vi "monitor scan logic.vi"(0 "Array IN":T4[](array[typedef]), 1 "monitor action":T3 caption="aaa", 2 "init":bool=TRUE, 5 "freq IN":dbl[](array[numeric]), 7 "Magn Field (T)":dbl, 9 "gamma IN":dbl[](array[numeric]), 11 "monitor state":T2={"header - gamma"=[], "header - frequency"=[], "# of peaks"=28, "peaks OK"=TRUE}, 12 "scan monitor control IN":T1={"gamma acc. frac. - min "=0.7, "gamma acc frac.. - max"=1.3, "peak acc. fraction (af)"=0.1, "min peak acc. window (kHz)"=0.1, "use"=enum."fraction", "abs gamma min(kHz)"=0.03, "abs gamma max(kHz)"=10.0, "# points"=0, "gamma-factor (fa)"=10.0, "interpolate"=enum."last", "init"=FALSE, "Unique strike parameters"=FALSE, "max peak acc. window (kHz)"=10.0, "spacing factor"=3.0, "iterate #"=1, "overwrite ctl?"=TRUE, "write _m files?"=FALSE, "max slope (kHz/sweep)"=0.1, "funnel state"=enum."funnel open"}, 13 "Sweep folder path":path=path "E:/data/Ultrasound/Experiment/ProbeTest/Probe10/Hg1201-350CO2-3b-96K/sweep2", 14 "temperature":dbl=309.595) -> (4 "Array OUT":T4[](array[typedef]), 6 "freq OUT":dbl[](array[numeric]), 10 "gamma OUT":dbl[](array[numeric]), 15 "monitor state OUT":T2={"header - gamma"=[], "header - frequency"=[], "# of peaks"=28, "peaks OK"=TRUE})   [LabVIEW 2015]
uses:
  peak monitor ctl - V2.ctl
  interpolation state - real.ctl
  parameters -- scan monitor control.ctl
  monitor action.ctl
  monitor state.ctl
  ctl -- name dispatcher -- action.ctl
  next chunk read-write PID -- action.ctl
  agregator -- action.ctl
  Q - not nan -- real.vi
  ctl -- name dispatcher.vi
  file -- 9w path.vi
  array -- find index - real.vi
  array -- interpolate -- i.vi
  Q - not nan -- integer.vi
  linear interpolation - real.vi
  <vilib>/gmath/function.llb/Binomial Coefficient.vi
  <vilib>/Utility/file.llb/Write To Spreadsheet File.vi
  <vilib>/Utility/file.llb/Write To Spreadsheet File (string).vi
  <vilib>/Utility/libraryn.llb/Check if File or Folder Exists.vi
  parse -- get list of matches -- numbers.vi
  parse -- find first line.vi
  file -- read list of lines.vi
panel:
  out "scan monitor control OUT":T1={"gamma acc. frac. - min "=0.7, "gamma acc frac.. - max"=1.3, "peak acc. fraction (af)"=0.1, "min peak acc. window (kHz)"=0.1, "use"=enum."fraction", "abs gamma min(kHz)"=0.03, "abs gamma max(kHz)"=10.0, "# points"=0, "gamma-factor (fa)"=10.0, "interpolate"=enum."last", "init"=FALSE, "Unique strike parameters"=FALSE, "max peak acc. window (kHz)"=10.0, "spacing factor"=3.0, "iterate #"=1, "overwrite ctl?"=TRUE, "write _m files?"=FALSE, "max slope (kHz/sweep)"=0.1, "funnel state"=enum."funnel open"}
  in  "Boolean":bool=TRUE
  # "three strikes"
  # "search window"
  # "linear extrapolation"
  # "three strikes"
  # "search window"
  # "linear extrapolation"
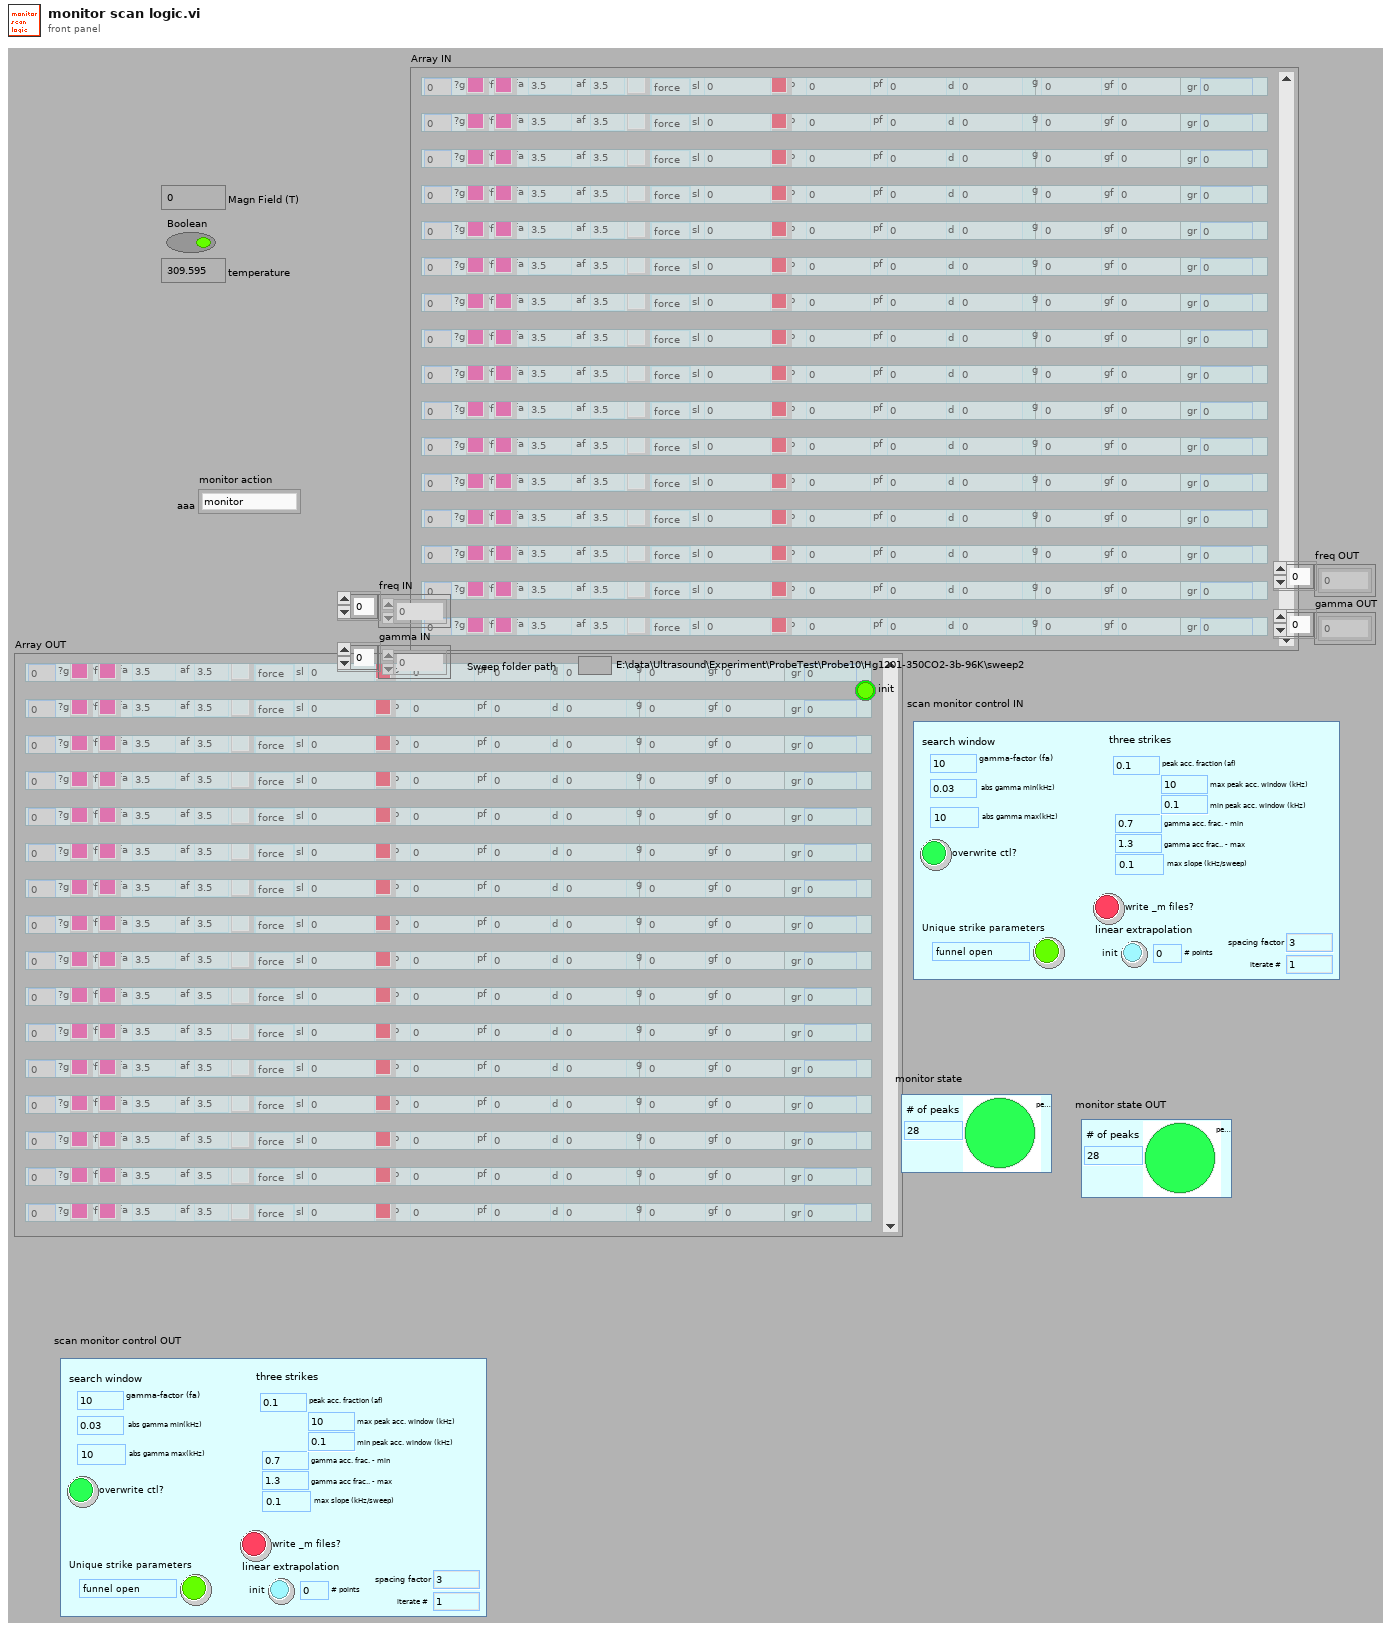
[diagram p1: front panel]
types:
  T1 = typedef "parameters -- scan monitor control.ctl" = cluster{"gamma acc. frac. - min ":dbl, "gamma acc frac.. - max":dbl, "peak acc. fraction (af)":dbl, "min peak acc. window (kHz)":dbl, "use":enum16{"window", "fraction"}, "abs gamma min(kHz)":dbl, "abs gamma max(kHz)":dbl, "# points":i32, "gamma-factor (fa)":dbl, "interpolate":enum16{"line", "last"}, "init":bool, "Unique strike parameters":bool, "max peak acc. window (kHz)":dbl, "spacing factor":dbl, "iterate #":i32, "overwrite ctl?":bool, "write _m files?":bool, "max slope (kHz/sweep)":dbl, "funnel state":enum16{"funnel open", "funnel closed"}}
  T2 = typedef "monitor state.ctl" = cluster{"header - gamma":string[], "header - frequency":string[], "# of peaks":i32, "peaks OK":bool}
  T3 = typedef "monitor action.ctl" = enum16{"monitor", "interpolate", "global", "read", "overwrite", "write m file", "nothing", "eeee"}
  T4 = typedef "peak monitor ctl - V2.ctl" = cluster{"delta":dbl, "gamma":dbl, "exp":dbl, "found?":bool, "found":dbl, "gamma found":dbl, "init linear":bool, "interpolate":enum16{"line", "force"}, "gamma-factor":dbl, "slope":dbl, "update freq?":bool, "update gamma?":bool, "acc factor":dbl, "linear interpolation state":T5, "ind":dbl, "gamma ratio":dbl, "gamma off limit?":bool, "freq off limit?":bool}
  T5 = typedef "interpolation state - real.ctl" = cluster{"requested size":i32, "Array":dbl[], "actual number of elements":i32}
  T6 = typedef "ctl -- name dispatcher -- action.ctl" = enum16{"peak frequency", "peak frequency DUMP", "peak gamma DUMP", "peak gamma", "peak frequency TEST", "peak gamma TEST", "ultrasonic power", "time in gamma", "set temperature ", "set temperature timer", "peak default gamma", "last scan file", "peak freq gamma TEST", "peak NAMES", "errors", "P_I_D", "P", "I", "D", "power vs time", "power vs time TIMER", "void", "power log", "set temperature - SINE", "itc ltc log", "peak - time in gamma"}
  T7 = typedef "agregator -- action.ctl" = enum16{"append", "interpolate", "empty!", "force"}
  T8 = typedef "next chunk read-write PID -- action.ctl" = enum16{"read", "interpolate", "append col", "write", "write PID col", "append PID col", "interpolate - bezier"}
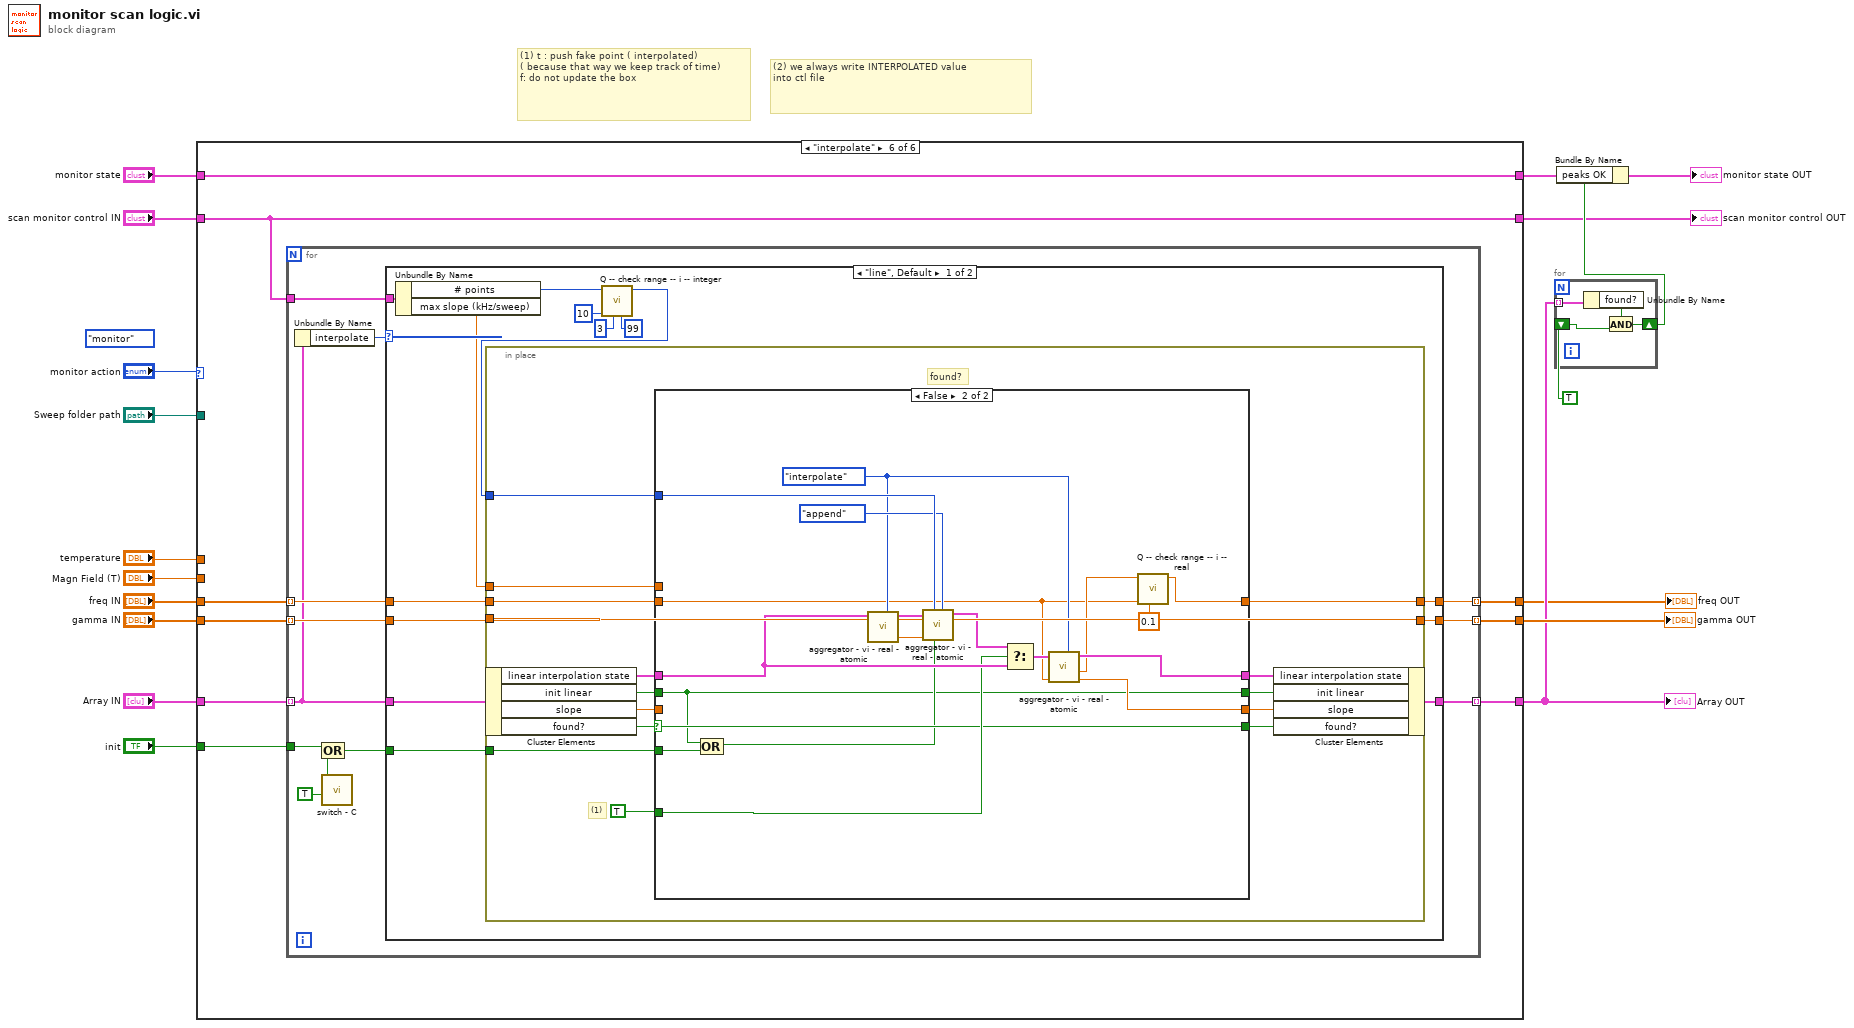
[diagram p0: block diagram]
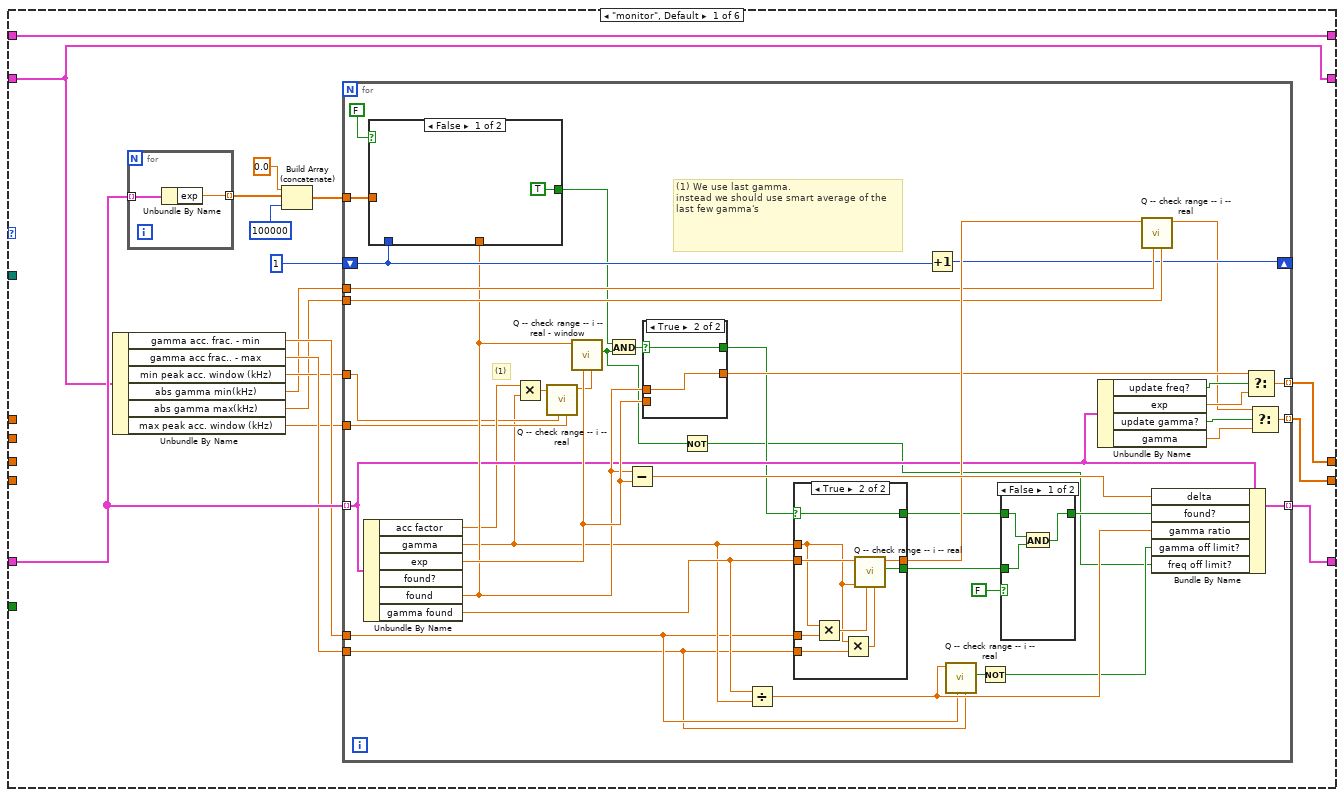
[diagram p2: hidden frame]
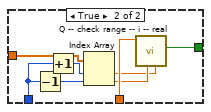
[diagram p3: hidden frame]
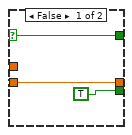
[diagram p6: hidden frame]
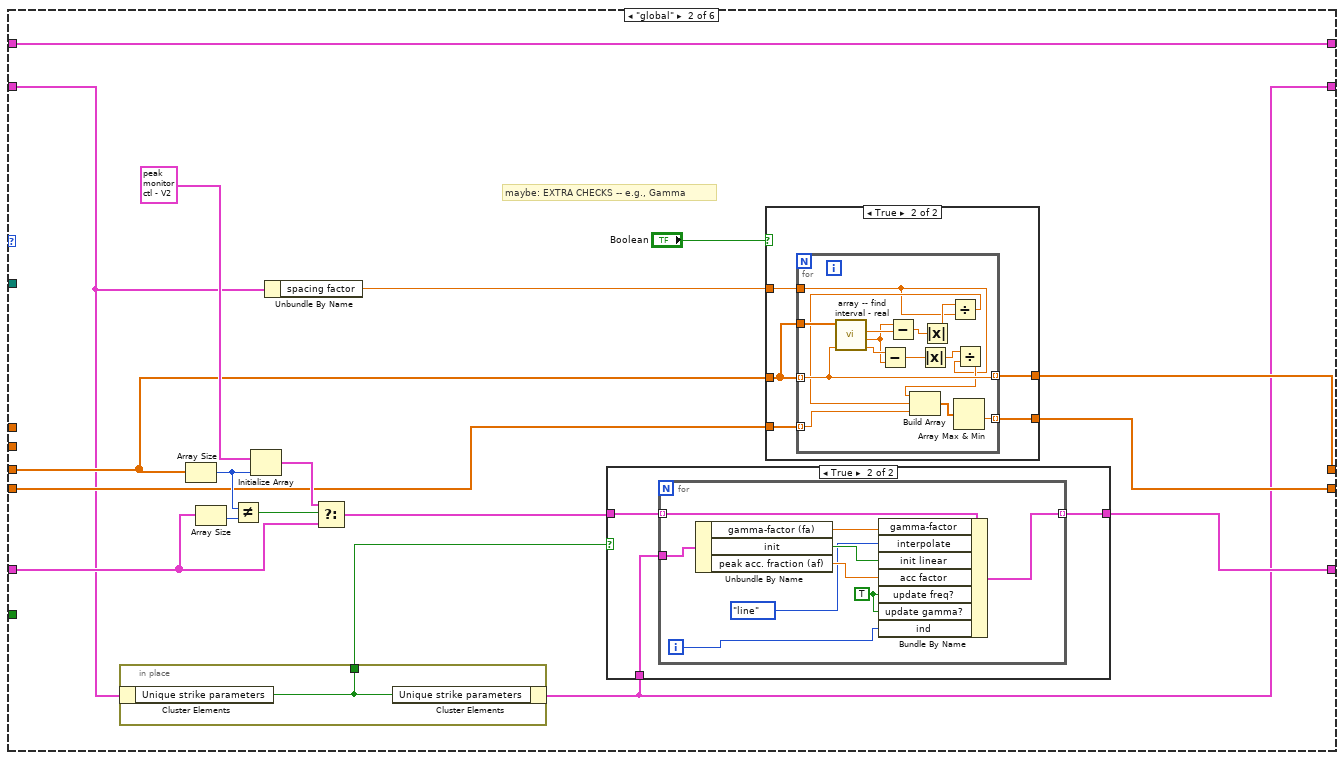
[diagram p7: hidden frame]
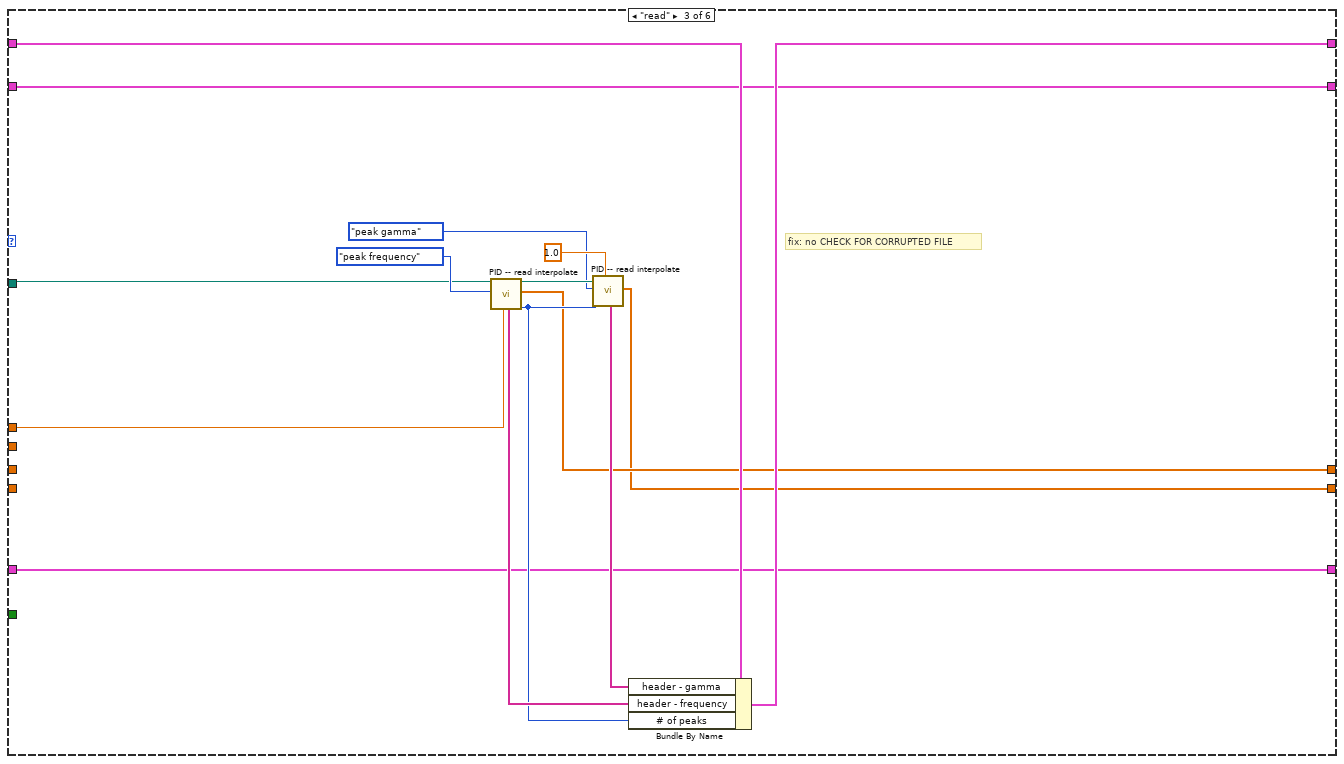
[diagram p10: hidden frame]
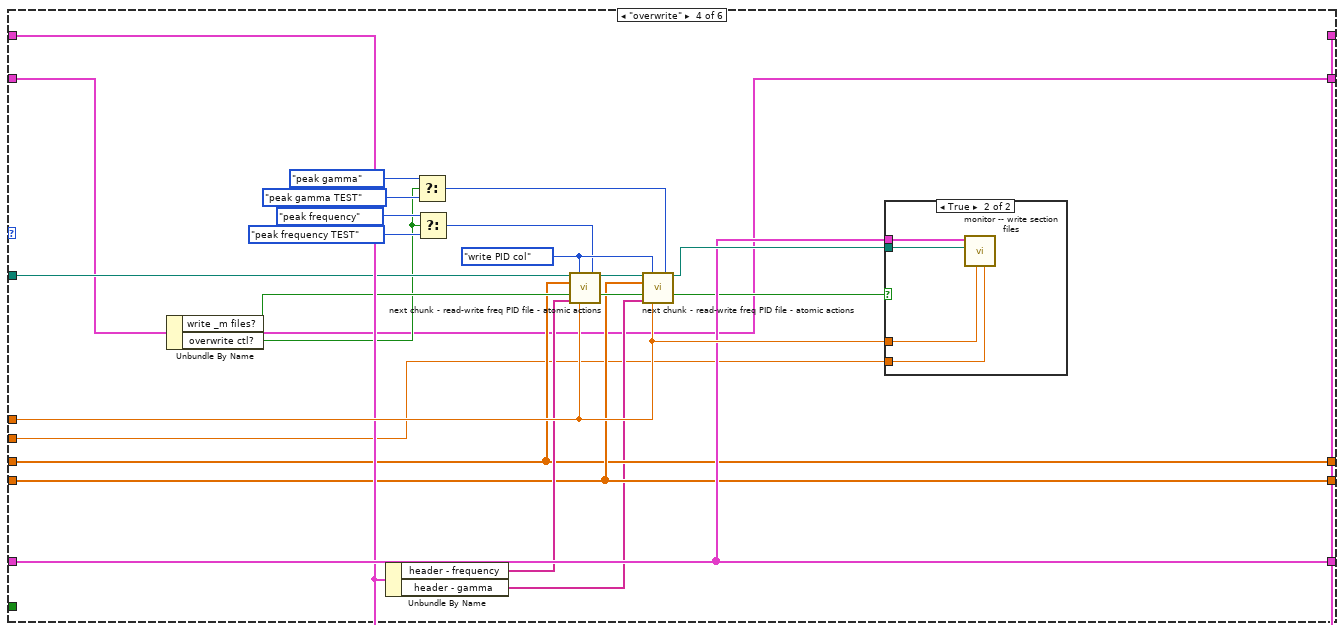
[diagram p11: hidden frame]
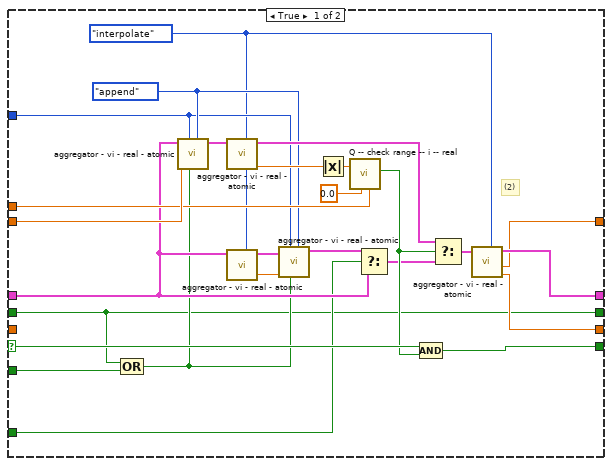
[diagram p14: hidden frame]
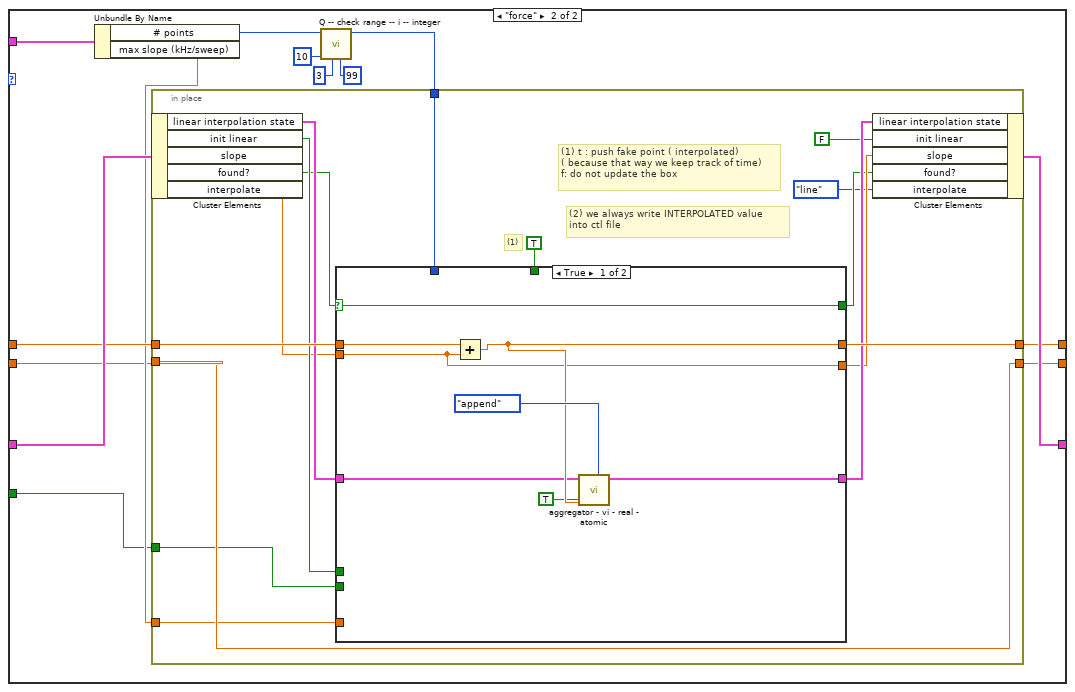
[diagram p15: hidden frame]
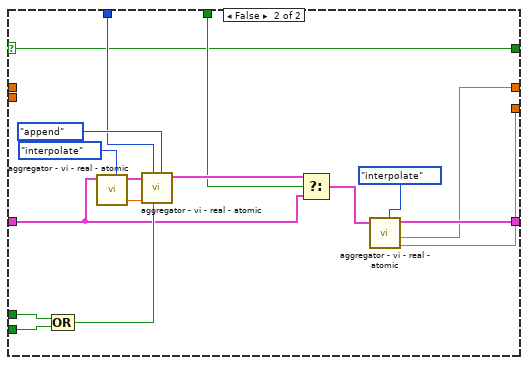
[diagram p16: hidden frame]
diagram:
  (unwired) monitor_action."monitor" ("monitor action")
  # "(2) we always write INTERPOLATED value \ninto ctl file"
  # "(1) t : push fake point ( interpolated) \n( because that way we keep track of time)\nf: do not update the box"
  n1 = case shown="\"interpolate\"" "monitor action" {
    tunnel: "scan monitor control IN" -> [w19 w109 w162 w177 w202 w207]
    tunnel: [w35 w115 w164 w180 w205 w214] -> w2
    tunnel: [w34 w114 w163 w181 w204 w212] -> w17
    tunnel: "Array IN" -> [w33 w119 w165 w187 w206 w215]
    tunnel: [w32 w125 w165 w187 w206 w210] -> w14
    tunnel: "freq IN" -> [_ w117 _ w180 w205 w213]
    tunnel: "gamma IN" -> [_ w116 _ w181 w204 w211]
    tunnel: "init" -> [_ _ _ _ _ w209]
    tunnel: "Sweep folder path" -> [_ _ w173 w184 _ _]
    tunnel: "temperature" -> [_ _ w172 w188 _ _]
    tunnel: "monitor state" -> [w20 w111 w170 w186 w203 w208]
    tunnel: [w20 w111 w167 w186 w203 w208] -> w5
    tunnel: "Magn Field (T)" -> [_ _ _ w178 _ _]
    tunnel: [w19 w108 w162 w177 w202 w207] -> w1
    frame "monitor", Default {
      n2 = Unbundle By Name(w19) -> ("gamma acc. frac. - min"=w31:dbl, "gamma acc frac.. - max"=w30:dbl, "min peak acc. window (kHz)"=w29:dbl, "abs gamma min(kHz)"=w28:dbl, "abs gamma max(kHz)"=w27:dbl, "max peak acc. window (kHz)"=w21:dbl)
      n3 = for {
        tunnel: w33 -> [w37] mode=indexing
        tunnel: [w36] -> w26 mode=indexing
        n4 = Unbundle By Name(w37) -> ("exp"=w36:dbl)
      }
      n5 = Build Array (concatenate)(0.0, w26, 100000) -> (w22:dbl[])
      n6 = for {
        tunnel: w33 -> [w66] mode=indexing
        tunnel: [w78] -> w32 mode=indexing
        tunnel: [w59] -> w34 mode=indexing
        tunnel: [w58] -> w35 mode=indexing
        tunnel: w31 -> [w44]
        tunnel: w30 -> [w43]
        tunnel: w29 -> [w56]
        tunnel: w28 -> [w75]
        tunnel: w27 -> [w74]
        shift-right: [w73] -> _
        shift-left: 1 -> [w72]
        tunnel: w22 -> [w71]
        tunnel: w21 -> [w55]
        # "(1)"
        # "(1) We use last gamma.\ninstead we should use smart average of the last few gamma's"
        n7 = Unbundle By Name(w66) -> ("acc factor"=w57:dbl, "gamma"=w46:dbl, "exp"=w69:dbl, "found"=w68:dbl, "gamma found"=w47:dbl)  [unwired: 1 out]
        n8 = case shown="False" FALSE ("in range?") {
          tunnel: w72 -> [_ w87]
          tunnel: w71 -> [_ w84]
          tunnel: w68 -> [_ w83]
          tunnel: [TRUE ("in range?") w80] -> w67
          frame False {
          }
          frame True {
            n9 = Decrement(x=w87) -> (x-1=w85:i32)
            n10 = Increment(x=w87) -> (x+1=w86:i32)
            n11 = Index Array(array=w84, index #1=w86, index #2=w85) -> (element #1=w81:dbl, element #2=w82:dbl)
            n12 = call "Q -- check range -- i -- real.vi"("upper"=w81, "lower"=w82, "number"=w83) -> ("in range?"=w80:bool)  [unwired: 6 in, 2 out]
          }
        }
        n13 = Multiply(x=w57, y=w46) -> (x*y=w54:dbl)
        n14 = call "Q -- check range -- i -- real.vi"("upper"=w55, "lower"=w56, "number"=w54) -> ("number in range"=w53:dbl)  [unwired: 6 in, 2 out]
        n15 = call "Q -- check range -- i -- real - window.vi"("window"=w53, "center"=w69, "number"=w68) -> ("in range?"=w40:bool)  [unwired: 6 in, 2 out]
        n16 = And(x=w67, y=w40) -> (x .and. y?=w70:bool)
        n17 = Subtract(x=w68, y=w69) -> (x-y=w77:dbl)
        n18 = case shown="True" w70 {
          selector: w70 -> [w92 w95]
          tunnel: [w92 w95] -> w52
          tunnel: [w93 w94] -> w64
          tunnel: w68 -> [_ w94]
          tunnel: w69 -> [w93 _]
          frame False {
          }
          frame True {
          }
        }
        n19 = Not(x=w40) -> (.not. x?=w39:bool)
        n20 = Divide(x=w47, y=w46) -> (x/y=w45:dbl)
        n21 = case shown="True" w52 {
          selector: w52 -> [w96 w99]
          tunnel: w47 -> [_ w107]
          tunnel: w46 -> [w98 w105]
          tunnel: [w98 w103] -> w76
          tunnel: w44 -> [_ w102]
          tunnel: w43 -> [_ w101]
          tunnel: [TRUE w100] -> w48
          tunnel: [w96 w99] -> w49
          frame False {
          }
          frame True {
            n22 = Multiply(x=w105, y=w102) -> (x*y=w106:dbl)
            n23 = Multiply(x=w105, y=w101) -> (x*y=w104:dbl)
            n24 = call "Q -- check range -- i -- real.vi"("upper"=w104, "lower"=w106, "default"=w105, "number"=w107) -> ("in range?"=w100:bool, "number in range"=w103:dbl)  [unwired: 5 in, 1 out]
          }
        }
        n25 = Increment(x=w72) -> (x+1=w73:i32)
        n26 = call "Q -- check range -- i -- real.vi"("upper"=w43, "lower"=w44, "number"=w45) -> ("in range?"=w42:bool)  [unwired: 6 in, 2 out]
        n27 = Not(x=w42) -> (.not. x?=w41:bool)
        n28 = case shown="False" FALSE {
          tunnel: [w88 w91] -> w50
          tunnel: w49 -> [w89 w91]
          tunnel: w48 -> [w90 _]
          frame False {
            n29 = And(x=w89, y=w90) -> (x .and. y?=w88:bool)
          }
          frame True {
          }
        }
        n30 = Unbundle By Name(w66) -> ("update freq?"=w65:bool, "exp"=w63:dbl, "update gamma?"=w62:bool, "gamma"=w60:dbl)
        n31 = call "Q -- check range -- i -- real.vi"("upper"=w74, "lower"=w75, "number"=w76) -> ("number in range"=w61:dbl)  [unwired: 6 in, 2 out]
        n32 = Bundle By Name(cluster=w66, "delta"=w77, "found?"=w50, "gamma ratio"=w45, "gamma off limit?"=w41, "freq off limit?"=w39) -> (w78:T4)
        n33 = Select(t=w64, s=w65, f=w63) -> (s? t:f=w58:dbl)
        n34 = Select(t=w61, s=w62, f=w60) -> (s? t:f=w59:dbl)
      }
    }
    frame "global" {
      # "maybe: EXTRA CHECKS -- e.g., Gamma"
      n35 = in-place {
        in-place-border: [w126] -> w110
        n36 = in-place-cluster #1(w109) -> ("Unique strike parameters"=w126:bool)
        n37 = in-place-cluster #1("Unique strike parameters"=w126) -> (w108:T1)
      }
      n38 = Array Size(array=w117) -> (size(s)=w123:i32)
      n39 = Array Size(array=w119) -> (size(s)=w124:i32)
      n40 = Not Equal?(x=w123, y=w124) -> (x != y?=w121:bool)
      n41 = Initialize Array(T4 {"delta"=0.0, "gamma"=0.0, "exp"=0.0, "found?"=FALSE, "found"=0.0, "gamma found"=0.0, "init linear"=FALSE, "interpolate"=enum."line", "gamma-factor"=0.0, "slope"=0.0, "update freq?"=FALSE, "update gamma?"=FALSE, "acc factor"=0.0, "linear interpolation state"={"requested size"=0, "Array"=[], "actual number of elements"=0}, "ind"=0.0, "gamma ratio"=0.0, "gamma off limit?"=FALSE, "freq off limit?"=FALSE} ("output cluster"), w123) -> (w120:T4[])
      n42 = Unbundle By Name(w109) -> ("spacing factor"=w112:dbl)
      n43 = Select(t=w120, s=w121, f=w119) -> (s? t:f=w118:T4[])
      n44 = case shown="True" w110 {
        tunnel: w118 -> [w149 w152]
        tunnel: [w149 w150] -> w125
        tunnel: w108 -> [_ w151]
        frame False {
        }
        frame True {
          n45 = for {
            tunnel: w152 -> [w156] mode=indexing
            tunnel: [w161] -> w150 mode=indexing
            tunnel: w151 -> [w160]
            i -> [w154]
            w155 = TRUE ("update freq?")
            n46 = Unbundle By Name(w160) -> ("gamma-factor (fa)"=w159:dbl, "init"=w158:bool, "peak acc. fraction (af)"=w157:dbl)
            n47 = Bundle By Name(cluster=w156, "gamma-factor"=w159, "interpolate"=enum16{"line", "force"}."line", "init linear"=w158, "acc factor"=w157, "update freq?"=w155, "update gamma?"=w155, "ind"=w154) -> (w161:T4)
          }
        }
      }
      n48 = case shown="True" "Boolean" {
        tunnel: w117 -> [w128 w133]
        tunnel: w116 -> [w127 w132]
        tunnel: [w128 w131] -> w115
        tunnel: [w127 w130] -> w114
        tunnel: w112 -> [_ w129]
        frame False {
        }
        frame True {
          n49 = for {
            tunnel: w133 -> [w144] mode=indexing
            tunnel: w133 -> [w148]
            tunnel: w132 -> [w141] mode=indexing
            tunnel: [w144] -> w131 mode=indexing
            tunnel: [w135] -> w130 mode=indexing
            tunnel: w129 -> [w134]
            n50 = call "array -- find interval - real.vi"("number"=w144, "array"=w148) -> ("omega plus (kHz)"=w146:dbl, "omega zero (kHz)"=w145:dbl, "omega minus (kHz)"=w147:dbl)  [unwired: 4 in, 3 out]
            n51 = Subtract(x=w146, y=w145) -> (x-y=w142:dbl)
            n52 = Subtract(x=w145, y=w147) -> (x-y=w143:dbl)
            n53 = Absolute Value(x=w142) -> (abs(x)=w139:dbl)
            n54 = Absolute Value(x=w143) -> (abs(x)=w140:dbl)
            n55 = Divide(x=w140, y=w134) -> (x/y=w137:dbl)
            n56 = Divide(x=w139, y=w134) -> (x/y=w138:dbl)
            n57 = Build Array(w138, w137, w141) -> (w136:dbl[])
            n58 = Array Max & Min(array=w136) -> (min value=w135:dbl)  [unwired: 3 out]
          }
        }
      }
    }
    frame "read" {
      # "fix: no CHECK FOR CORRUPTED FILE"
      n59 = call "PID -- read interpolate.vi"("sweep folder path"=w173, "ctl PID file IN"=ctl_--_name_dispatcher_--_action."peak frequency" ("ctl name dispatch"), "temperature"=w172) -> ("header"=w168:string[], "sweep folder path out"=w175:path, "PID freq"=w164:dbl[], "length out"=w166:i32)  [unwired: 11 in, 2 out]
      n60 = call "PID -- read interpolate.vi"("sweep folder path"=w175, "ctl PID file IN"=ctl_--_name_dispatcher_--_action."peak gamma" ("ctl name dispatch"), "length"=w166, "default"=1.0 ("element")) -> ("header"=w169:string[], "PID freq"=w163:dbl[])  [unwired: 10 in, 4 out]
      n61 = Bundle By Name(cluster=w170, "header - gamma"=w169, "header - frequency"=w168, "# of peaks"=w166) -> (w167:T2)
    }
    frame "overwrite" {
      w196 = next_chunk_read-write_PID_--_action."write PID col" ("PID action")
      n62 = Unbundle By Name(w177) -> ("write _m files?"=w183:bool, "overwrite ctl?"=w182:bool)
      n63 = Unbundle By Name(w186) -> ("header - frequency"=w185:string[], "header - gamma"=w179:string[])
      n64 = Select(t=ctl_--_name_dispatcher_--_action."peak gamma" ("ctl name dispatch"), s=w182, f=ctl_--_name_dispatcher_--_action."peak gamma TEST" ("ctl name dispatch")) -> (s? t:f=w195:T6)
      n65 = Select(t=ctl_--_name_dispatcher_--_action."peak frequency" ("ctl name dispatch"), s=w182, f=ctl_--_name_dispatcher_--_action."peak frequency TEST" ("ctl name dispatch")) -> (s? t:f=w194:T6)
      n66 = call "next chunk - read-write freq PID file - atomic actions .vi"("sweep folder path"=w184, "PID action"=w196, "ctl kind OUT"=w194, "PID freq IN"=w180, "header IN"=w185, "temperature"=w188) -> ("sweep folder path out"=w197:path)  [unwired: 5 in, 4 out]
      n67 = call "next chunk - read-write freq PID file - atomic actions .vi"("sweep folder path"=w197, "PID action"=w196, "ctl kind OUT"=w195, "PID freq IN"=w181, "header IN"=w179, "temperature"=w188) -> ("sweep folder path out"=w193:path)  [unwired: 5 in, 4 out]
      n68 = case shown="True" w183 {
        tunnel: w193 -> [_ w201]
        tunnel: w187 -> [_ w200]
        tunnel: w188 -> [_ w199]
        tunnel: w178 -> [_ w198]
        frame False {
        }
        frame True {
          n69 = call "monitor -- write section files.vi"("Magn Field (T)"=w198, "temperature"=w199, "Sweep folder path"=w201, "Array"=w200) -> ()  [unwired: 8 in]
        }
      }
    }
    frame "nothing" {
    }
    frame "interpolate" {
      n70 = for {
        tunnel: w215 -> [w221] mode=indexing
        tunnel: [w226] -> w214 mode=indexing
        tunnel: w213 -> [w225] mode=indexing
        tunnel: [w224] -> w212 mode=indexing
        tunnel: w211 -> [w223] mode=indexing
        tunnel: [w222] -> w210 mode=indexing
        tunnel: w209 -> [w218]
        tunnel: w207 -> [w220]
        n71 = Unbundle By Name(w221) -> ("interpolate"=w227:enum16{"line", "force"})
        n72 = call "switch - C.vi"("switch"=TRUE) -> ("result"=w216:bool)  [unwired: 10 in]
        n73 = Compound Arithmetic op=OR(w218, w216) -> (w217:bool)
        n74 = case shown="\"line\", Default" w227 {
          tunnel: [w232 w306] -> w226
          tunnel: w225 -> [w234 w308]
          tunnel: [w230 w304] -> w224
          tunnel: w223 -> [w231 w305]
          tunnel: [w235 w309] -> w222
          tunnel: w221 -> [w236 w310]
          tunnel: w220 -> [w237 w311]
          tunnel: w217 -> [w228 w302]
          frame "line", Default {
            n75 = Unbundle By Name(w237) -> ("# points"=w238:i32, "max slope (kHz/sweep)"=w233:dbl)
            n76 = call "Q -- check range -- i -- integer.vi"("upper"=99, "lower"=3, "default"=10, "number"=w238) -> ("number in range"=w229:i32)  [unwired: 5 in, 2 out]
            n77 = in-place {
              in-place-border: w234 -> [w255]
              in-place-border: w228 -> [w253]
              in-place-border: w233 -> [w249]
              in-place-border: [w254] -> w232
              in-place-border: w231 -> [w256]
              in-place-border: [w256] -> w230
              in-place-border: w229 -> [w252]
              # "found?"
              # "(1)"
              n78 = in-place-cluster #2(w236) -> ("linear interpolation state"=w251:T5, "init linear"=w242:bool, "slope"=w244:dbl, "found?"=w247:bool)
              n79 = case shown="False" w247 {
                selector: w247 -> [w271 w295]
                tunnel: w255 -> [w281 w283]
                tunnel: [w260 w284] -> w254
                tunnel: w253 -> [w282 w301]
                tunnel: w252 -> [w266 w298]
                tunnel: w251 -> [w262 w297]
                tunnel: [w273 w300] -> w250
                tunnel: w249 -> [w276 _]
                tunnel: [w272 w299] -> w248
                tunnel: [w269 w295] -> w246
                tunnel: TRUE ("s") -> [w261 w296]
                tunnel: w244 -> [_ _]
                tunnel: [w258 w293] -> w243
                tunnel: w242 -> [w258 w293]
                frame True {
                  w257 = agregator_--_action."interpolate" ("aggregator action")
                  w267 = agregator_--_action."append" ("aggregator action")
                  # "(2)"
                  n80 = Compound Arithmetic op=OR(w258, w282) -> (w259:bool)
                  n81 = call "aggregator - vi - real - atomic.vi"("aggregator action"=w267, "init?"=w259, "requested size"=w266, "number"=w281, "state IN"=w262) -> ("state OUT"=w280:T5)  [unwired: 3 in, 3 out]
                  n82 = call "aggregator - vi - real - atomic.vi"("aggregator action"=w257, "state IN"=w280) -> ("slope"=w277:dbl, "state OUT"=w275:T5)  [unwired: 6 in, 2 out]
                  n83 = call "aggregator - vi - real - atomic.vi"("aggregator action"=w257, "state IN"=w262) -> ("interp average"=w265:dbl, "state OUT"=w268:T5)  [unwired: 6 in, 2 out]
                  n84 = call "aggregator - vi - real - atomic.vi"("aggregator action"=w267, "init?"=w259, "requested size"=w266, "number"=w265, "state IN"=w268) -> ("state OUT"=w264:T5)  [unwired: 3 in, 3 out]
                  n85 = Absolute Value(x=w277) -> (abs(x)=w279:dbl)
                  n86 = call "Q -- check range -- i -- real.vi"("upper"=w276, "lower"=0.0, "number"=w279) -> ("in range?"=w270:bool)  [unwired: 6 in, 2 out]
                  n87 = Select(t=w264, s=w261, f=w262) -> (s? t:f=w263:T5)
                  n88 = Compound Arithmetic op=AND(w271, w270) -> (w269:bool)
                  n89 = Select(t=w275, s=w270, f=w263) -> (s? t:f=w274:T5)
                  n90 = call "aggregator - vi - real - atomic.vi"("aggregator action"=w257, "state IN"=w274) -> ("slope"=w272:dbl, "interp average"=w260:dbl, "state OUT"=w273:T5)  [unwired: 6 in, 1 out]
                }
                frame False {
                  w287 = agregator_--_action."interpolate" ("aggregator action")
                  n91 = Compound Arithmetic op=OR(w293, w301) -> (w294:bool)
                  n92 = call "aggregator - vi - real - atomic.vi"("aggregator action"=w287, "state IN"=w297) -> ("interp average"=w290:dbl, "state OUT"=w292:T5)  [unwired: 6 in, 2 out]
                  n93 = call "aggregator - vi - real - atomic.vi"("aggregator action"=agregator_--_action."append", "init?"=w294, "requested size"=w298, "number"=w290, "state IN"=w292) -> ("state OUT"=w289:T5)  [unwired: 3 in, 3 out]
                  n94 = Select(t=w289, s=w296, f=w297) -> (s? t:f=w288:T5)
                  n95 = call "aggregator - vi - real - atomic.vi"("aggregator action"=w287, "number"=w283, "state IN"=w288) -> ("slope"=w299:dbl, "interp average"=w285:dbl, "state OUT"=w300:T5)  [unwired: 5 in, 1 out]
                  n96 = call "Q -- check range -- i -- real.vi"("lower"=0.1, "default"=w283, "number"=w285) -> ("number in range"=w284:dbl)  [unwired: 6 in, 2 out]
                }
              }
              n97 = in-place-cluster #2("linear interpolation state"=w250, "init linear"=w243, "slope"=w248, "found?"=w246) -> (w235:T4)
            }
          }
          frame "force" {
            n98 = Unbundle By Name(w311) -> ("# points"=w312:i32, "max slope (kHz/sweep)"=w307:dbl)
            n99 = call "Q -- check range -- i -- integer.vi"("upper"=99, "lower"=3, "default"=10, "number"=w312) -> ("number in range"=w303:i32)  [unwired: 5 in, 2 out]
            n100 = in-place {
              in-place-border: w308 -> [w330]
              in-place-border: w302 -> [w328]
              in-place-border: w307 -> [w323]
              in-place-border: [w329] -> w306
              in-place-border: w305 -> [w331]
              in-place-border: [w331] -> w304
              in-place-border: w303 -> [w326]
              # "(2) we always write INTERPOLATED value \ninto ctl file"
              # "(1)"
              # "(1) t : push fake point ( interpolated) \n( because that way we keep track of time)\nf: do not update the box"
              n101 = in-place-cluster #3(w310) -> ("linear interpolation state"=w325:T5, "init linear"=w327:bool, "slope"=w318:dbl, "found?"=w321:bool)  [unwired: 1 out]
              n102 = case shown="True" w321 {
                selector: w321 -> [w332 w341]
                tunnel: w330 -> [w338 _]
                tunnel: [w337 w340] -> w329
                tunnel: w328 -> [_ w356]
                tunnel: w327 -> [_ w355]
                tunnel: w326 -> [_ w348]
                tunnel: w325 -> [w335 w344]
                tunnel: [w334 w353] -> w324
                tunnel: w323 -> [_ _]
                tunnel: [w333 w352] -> w322
                tunnel: [w332 w341] -> w320
                tunnel: TRUE ("s") -> [_ w343]
                tunnel: w318 -> [w333 _]
                frame True {
                  n103 = Add(x=w338, y=w333) -> (x+y=w337:dbl)
                  n104 = call "aggregator - vi - real - atomic.vi"("aggregator action"=agregator_--_action."append", "init?"=TRUE, "number"=w337, "state IN"=w335) -> ("state OUT"=w334:T5)  [unwired: 4 in, 3 out]
                }
                frame False {
                  n105 = Compound Arithmetic op=OR(w355, w356) -> (w346:bool)
                  n106 = call "aggregator - vi - real - atomic.vi"("aggregator action"=agregator_--_action."interpolate", "state IN"=w344) -> ("interp average"=w347:dbl, "state OUT"=w350:T5)  [unwired: 6 in, 2 out]
                  n107 = call "aggregator - vi - real - atomic.vi"("aggregator action"=agregator_--_action."append", "init?"=w346, "requested size"=w348, "number"=w347, "state IN"=w350) -> ("state OUT"=w345:T5)  [unwired: 3 in, 3 out]
                  n108 = Select(t=w345, s=w343, f=w344) -> (s? t:f=w342:T5)
                  n109 = call "aggregator - vi - real - atomic.vi"("aggregator action"=agregator_--_action."interpolate", "state IN"=w342) -> ("slope"=w352:dbl, "interp average"=w340:dbl, "state OUT"=w353:T5)  [unwired: 6 in, 1 out]
                }
              }
              n110 = in-place-cluster #3("linear interpolation state"=w324, "init linear"=FALSE, "slope"=w322, "found?"=w320, "interpolate"=enum16{"line", "force"}."line") -> (w309:T4)
            }
          }
        }
      }
    }
  }
  "freq OUT" <- w2
  "gamma OUT" <- w17
  "Array OUT" <- w14
  "scan monitor control OUT" <- w1
  n111 = for {
    tunnel: w14 -> [w360] mode=indexing
    shift-right: [w359] -> w6
    shift-left: TRUE -> [w357]
    n112 = Unbundle By Name(w360) -> ("found?"=w358:bool)
    n113 = And(x=w358, y=w357) -> (x .and. y?=w359:bool)
  }
  n114 = Bundle By Name(cluster=w5, "peaks OK"=w6) -> (→"monitor state OUT":T2)
